vi "JAUS Set Target Loop.vi"() -> ()   [LabVIEW 2009]
uses:
  JAUS/Support Files/LocalPose.ctl
  JAUS/Support Files/TimeRec.ctl
  <vilib>/Platform/TimedLoop/XDataNode/XDataNode.xnode
  <vilib>/Platform/TimedLoop/XDataNode/loadlvalarms.vi
  <vilib>/Platform/TimedLoop/XDataNode/timing_clust.ctl
  <vilib>/Platform/TimedLoop/XDataNode/nitl_modes.ctl
  <vilib>/Platform/TimedLoop/XDataNode/wakeup.ctl
  Functional Global Variables/Actions for FG's.ctl
  <vilib>/Platform/TimedLoop/XDataNode/XDNodeRunTimeDep.lvlib
panel:
  in  "LocalPose":T1
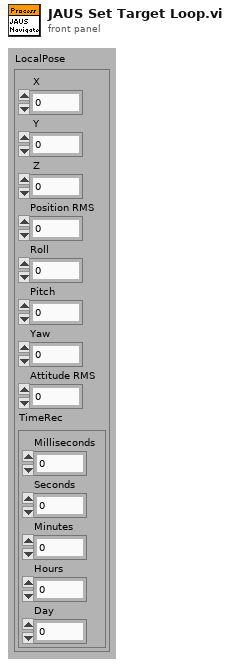
[diagram p1: front panel]
types:
  T1 = typedef "LocalPose.ctl" = cluster{" X":dbl, " Y":dbl, " Z":dbl, "Position RMS":dbl, "Roll":dbl, "Pitch":dbl, "Yaw":dbl, "Attitude RMS":dbl, "TimeRec":T2}
  T2 = typedef "TimeRec.ctl" = cluster{"Milliseconds":u32, "Seconds":u32, "Minutes":u32, "Hours":u32, "Day":u32}
  T3 = typedef "XDNodeRunTimeDep.lvlib/timing_clust.ctl" = cluster{"Expected End [f-1]":u64, "Actual End [f-1]":u64, "Finished Late? [f-1]":bool, "Expected End [i-1]":u64, "Actual End [i-1]":u64, "Finished Late? [i-1]":bool, "Expected Start [i]":u64, "Actual Start [i]":u64, "Expected Start [f]":u64, "Actual Start [f]":u64, "Source Name":string, "Structure Name":string, "Period":i64, "Deadline":i64, "Offset":i64, "Start":i64, "Priority":i32, "Timeout":i32, "Mode":T4, "Wakeup Reason":T5, "Error":errorcluster, "Source Type":string, "Secondary Source Type":string, "Global End Time":u64, "Global Start Time":u64, "Frame Duration":u64, "Iteration Duration":u64, "Assigned CPU":i32, "I/O Scan Engine Mode":u32}
  T4 = typedef "XDNodeRunTimeDep.lvlib/nitl_modes.ctl" = enum32{"No Change", "Process missed periods, maintain original phase", "Discard missed periods, maintain original phase", "Process missed periods, ignore original phase", "Discard missed periods, ignore original phase"}
  T5 = typedef "XDNodeRunTimeDep.lvlib/wakeup.ctl" = enum32{"Normal", "Aborted", "Asynchronous wakeup", "Timing source error", "Timed loop error", "Timeout"}
  T6 = typedef "Actions for FG's.ctl" = enum16{"Read", "Write"}
  T7 = typedef "GPS Data.ctl" = cluster{"Latitude":dbl, "Longitude":dbl}
  T8 = typedef "ElementRec.ctl" = cluster{"ElementUID":u16, " PreviousUID":u16, " NextUID":u16, "LocalWaypointRec":T9}
  T9 = typedef "LocalWaypointRec.ctl" = cluster{"Presence Vector":u8, " X":dbl, " Y":dbl, " Z":dbl, "Roll":dbl, "Pitch":dbl, "Yaw":dbl, "Waypoint Tolerance":dbl, "Path Tolerance":dbl, "Is Active?":bool}
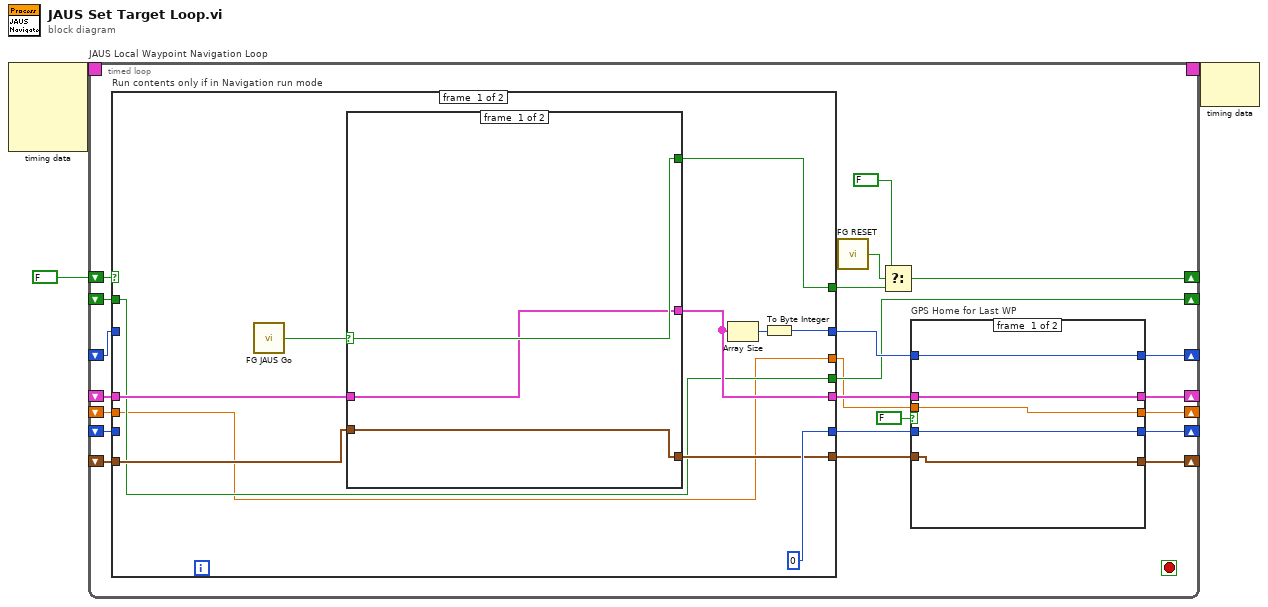
[diagram p0: block diagram]
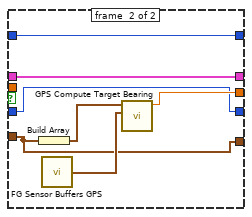
[diagram p2: hidden frame]
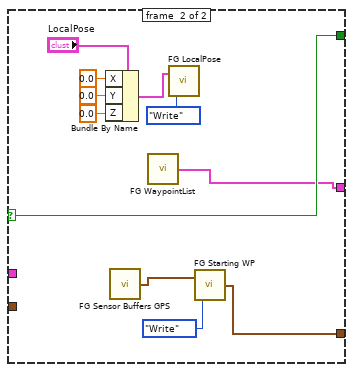
[diagram p3: hidden frame]
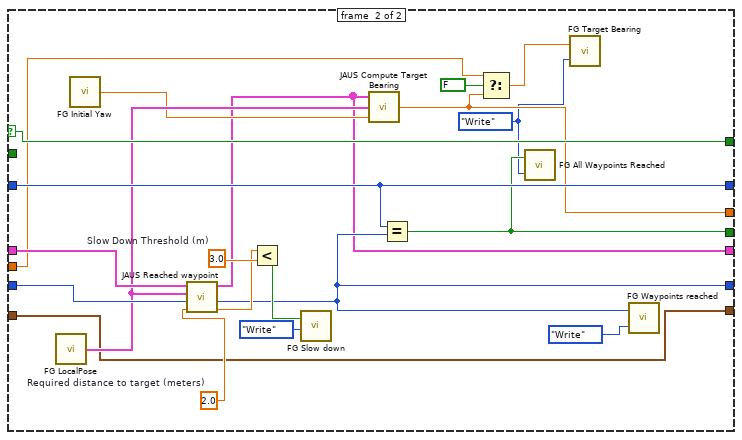
[diagram p4: hidden frame]
diagram:
  n1 = node-c288() -> (w3:T3)  [unwired: 4 in]
  n2 = timed-loop "JAUS Local Waypoint Navigation Loop" {
    timing: w3 -> [_]
    timing-out: [_] -> w2
    shift-right: [w12] -> _
    shift-left: _ -> [w26]
    shift-right: [w14] -> _
    shift-left: _ -> [w24]
    shift-right: [w20] -> _
    shift-left: FALSE ("t") -> [w19]
    shift-right: [w16] -> _
    shift-left: _ -> [w25]
    shift-right: [w10] -> _
    shift-left: _ -> [w18]
    shift-right: [w9] -> _
    shift-left: _ -> [w8]
    shift-right: [w7] -> _
    shift-left: _ -> [w6]
    stop <- _ stop-if-true
    n3 = case "Run contents only if in Navigation run mode" shown="True" w19 {
      selector: w19 -> [_ w82]
      tunnel: w26 -> [_ w76]
      tunnel: w25 -> [_ w81]
      tunnel: [i8 0 ("Number of WP Reached OUT") w75] -> w13
      tunnel: w24 -> [w47 w84]
      tunnel: [w45 w71] -> w15
      tunnel: [w49 w82] -> w21
      tunnel: [w39 w81] -> w17
      tunnel: [w43 w65] -> w11
      tunnel: w18 -> [w42 w65]
      tunnel: [w41 w70] -> w9
      tunnel: w8 -> [w41 _]
      tunnel: [w40 w68] -> w5
      tunnel: w6 -> [w40 w69]
      frame #0 {
        n4 = call "FG JAUS Go.vi"() -> ("Go Out"=w44:bool)  [unwired: 2 in]
        n5 = case shown="False" w44 {
          selector: w44 -> [w52 w63]
          tunnel: [w52 w63] -> w49
          tunnel: w47 -> [w51 _]
          tunnel: [w51 w62] -> w45
          tunnel: [w50 w54] -> w43
          tunnel: w42 -> [w50 _]
          frame #0 {
          }
          frame #1 {
            n6 = Bundle By Name(cluster="LocalPose", "X"=0.0, "Y"=0.0, "Z"=0.0) -> (w60:T1)
            n7 = call "FG Sensor Buffers GPS.vi"() -> ("GPS Buffer out"=w55:T7)  [unwired: 2 in]
            n8 = call "FG WaypointList.vi"() -> ("Local Waypoint List out"=w62:T8[])  [unwired: 2 in]
            n9 = call "FG LocalPose.vi"("FG Action (Read)"=Actions_for_FG's."Write", "LocalPose in"=w60) -> ()  [unwired: 1 out]
            n10 = call "FG Starting WP.vi"("FG Action (Read)"=Actions_for_FG's."Write", "Starting WP in"=w55) -> ("Starting WP out"=w54:T7)
          }
        }
        n11 = Array Size(array=w45) -> (size(s)=w48:i32)
        n12 = To Byte Integer(number=w48) -> (8bit integer=w39:i8)
      }
      frame #1 {
        w80 = 3.0  # Slow Down Threshold (m)
        w66 = Actions_for_FG's."Write" ("FG Action (Read)")
        w74 = 2.0  # Required distance to target (meters)
        n13 = call "FG LocalPose.vi"() -> ("LocalPose out"=w73:T1)  [unwired: 2 in]
        n14 = call "FG Initial Yaw.vi"() -> ("Initial Yaw Out"=w72:dbl)  [unwired: 2 in]
        n15 = call "JAUS Reached waypoint.vi"("Required distance to target (meters)"=w74, "Number of WP Reached IN"=w76, "LocalPose in"=w73, "Local Waypoint List in"=w84) -> ("Distance to Target (meters)"=w77:dbl, "Number of WP Reached OUT"=w75:i8, "Local Waypoint List Out"=w71:T8[])  [unwired: 4 in, 1 out]
        n16 = Less?(x=w77, y=w80) -> (x < y?=w79:bool)
        n17 = call "FG Slow down.vi"("FG Action (Read)"=Actions_for_FG's."Write", "Slow down in"=w79) -> ()  [unwired: 1 out]
        n18 = call "JAUS Compute Target Bearing.vi"("Initial Yaw In"=w72, "LocalPose in"=w73, "Local Waypoint List Out"=w71) -> ("Target Bearing (Yaw) (degrees)"=w68:dbl)
        n19 = Equal?(x=w81, y=w75) -> (x = y?=w70:bool)
        n20 = Select(t=w69, s=FALSE, f=w68) -> (s? t:f=w67:dbl)
        n21 = call "FG All Waypoints Reached.vi"("FG Action (Read)"=w66, "All waypoints reached in"=w70) -> ()  [unwired: 1 in, 1 out]
        n22 = call "FG Target Bearing.vi"("FG Action (Read)"=w66, "Target Bearing in"=w67) -> ()  [unwired: 1 out]
        n23 = call "FG Waypoints reached.vi"("FG Action (Read)"=Actions_for_FG's."Write", "Waypoints reached in"=w75) -> ()  [unwired: 1 in, 1 out]
      }
    }
    n24 = call "FG RESET.vi"() -> ("RESET out"=w23:bool)  [unwired: 2 in]
    n25 = Select(t=FALSE, s=w23, f=w21) -> (s? t:f=w20:bool)
    n26 = case "GPS Home for Last WP" shown="False" FALSE {
      tunnel: w17 -> [w31 w35]
      tunnel: [w31 w35] -> w16
      tunnel: w15 -> [w30 w34]
      tunnel: [w30 w34] -> w14
      tunnel: w13 -> [w29 w32]
      tunnel: [w29 w32] -> w12
      tunnel: w11 -> [w28 w33]
      tunnel: [w28 w33] -> w10
      tunnel: [w27 w36] -> w7
      tunnel: w5 -> [w27 _]
      frame #0 {
      }
      frame #1 {
        n27 = Build Array(w33) -> (w38:T7[])
        n28 = call "FG Sensor Buffers GPS.vi"() -> ("GPS Buffer out"=w37:T7)  [unwired: 2 in]
        n29 = call "GPS Compute Target Bearing.vi"("Current co-ordinates"=w37, "GPS Waypoint List Out"=w38) -> ("Target Bearing (degrees)"=w36:dbl)  [unwired: 8 in]
      }
    }
  }
  n30 = node-c288(w2) -> ()  [unwired: 1 out]
